vi "Test_Install_IPK.vi"(4 "error in":errorcluster, 7 "Parameter Array in":string[](array[string])) -> (0 "error out":errorcluster, 1 "Result Paragraphs":string[](array[string]), 2 "Pass":bool, 3 "Parameter Array Out":string[](array[string]))   [LabVIEW 2020]
uses:
  <vilib>/nisyscfg/Software 1.2.ctl
  <vilib>/nisyscfg/Component Type.ctl
  CommonSubVIs/Framework/Flattened_Array/Test Parameter Enum.ctl
  CommonSubVIs/Framework/Flattened_Array/Get Parameter Value by Name (String).vi
  <vilib>/nisyscfg/Get Installed Components.vi
  <vilib>/nisyscfg/Close (System).vi
  <resource>/objmgr/nisysapi.rc
  <vilib>/nisyscfg/nisyscfg.lvlib
panel:
  out "Greenways\nBoolean":bool
  in  "Tab Control":T1(tab)
  in  "Network Address":string="10.0.62.162"
  out "Format Python result":string
  out "Format Return Code":i32
  out "Format\nBoolean":bool
  out "Setup Python result":string
  out "Setup Return Code":i32
  out "Setup\nBoolean":bool
  out "GreenWays Python result":string
  out "Greenways Return Code":i32
  out "Installed Software 1":T2[](array[typedef]) caption="Installed Software" {"component type" items=["standard", "hidden", "system", "unknown", "startup", "image", "essential"]}
  # "This VI is used to Format For IPK installation Using python script."
  # "This VI is used to install SetupLinux for RT IPK  Using python script."
  # "This VI is used to install Greenway and FTP software to the (IPK) Linux target Using python script."
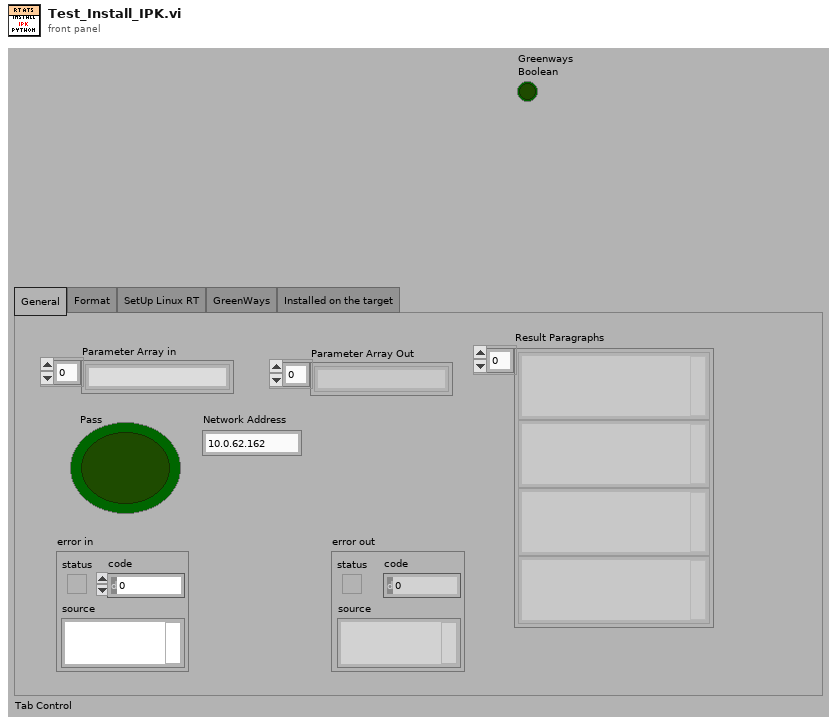
[diagram p1: front panel]
types:
  T1 = enum32{"General", "Format", "SetUp Linux RT", "GreenWays", "Installed on the target"}
  T2 = typedef "nisyscfg.lvlib/Software 1.2.ctl" = cluster{"title":string, "description":string, "ID":string, "version":string, "component type":T3}
  T3 = typedef "nisyscfg.lvlib/Component Type.ctl" = u32
  T4 = typedef "Test Parameter Enum.ctl" = enum16{"Main Test Target IP", "Main Test Target Name", "Main Test Target Alias", "Main Host IP", "Default Target Alias", "Default Target Host Name", "Dafault Target IP Address", "Dafault Target LV Date", "Available Targets", "Target Alias by Index", "Target IP by Alias", "Target IP by  Index", "Current Iteration", "Total Iterations", "Test Project Name", "Current Test Result", "Current Test Name", "Current Test Logical Path", "Test Folder", "Configuration Name", "Configuration Index", "Total Configurations", "Performance Values", "Result Paragraphs", "Connector Pane", "Avoid?", "Avoid Reason", "Case Name", "Case #", "Total Cases", "Case Data", "Disable reason"}
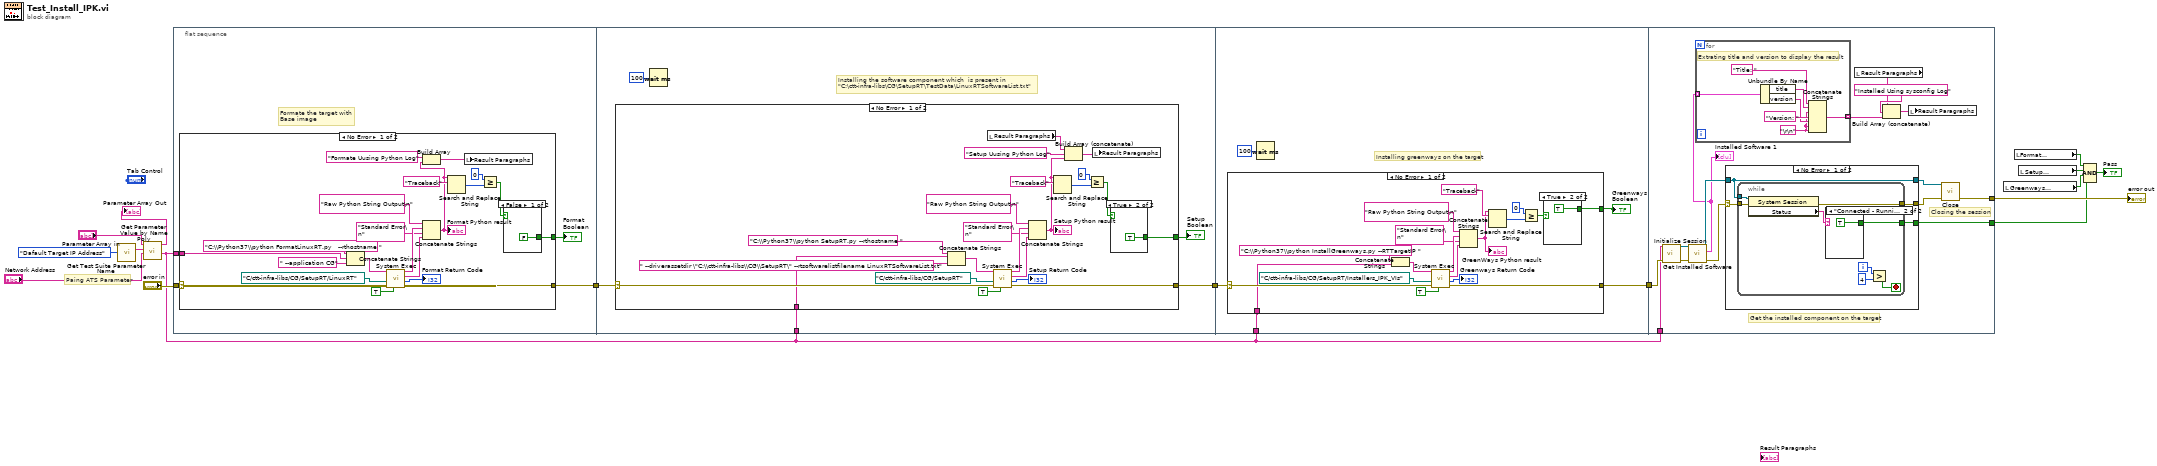
[diagram p0: block diagram]
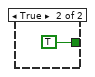
[diagram p2: hidden frame]
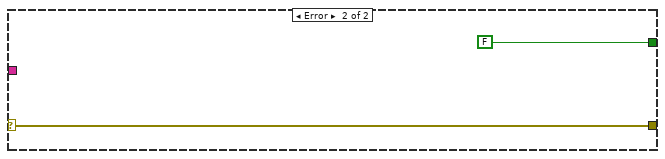
[diagram p3: hidden frame]
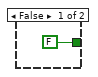
[diagram p4: hidden frame]
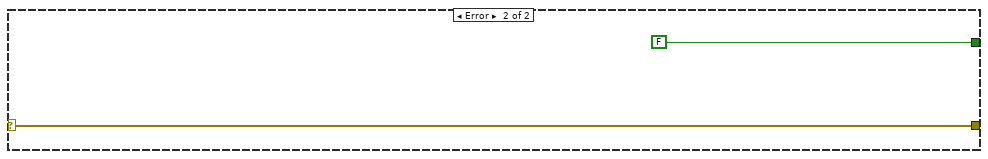
[diagram p5: hidden frame]
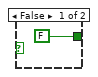
[diagram p6: hidden frame]
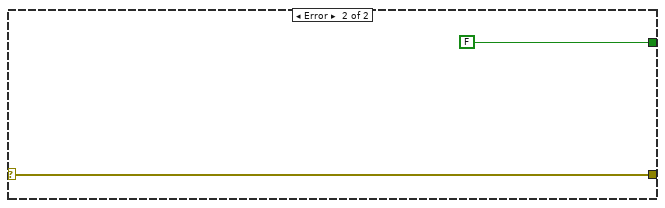
[diagram p7: hidden frame]
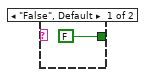
[diagram p8: hidden frame]
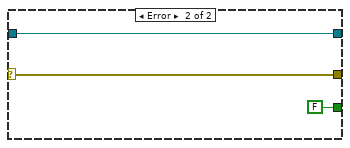
[diagram p9: hidden frame]
diagram:
  # "Paing ATS Parameter"
  n1 = call "Get Test Suite Parameter Name.vi"("Test Suite Parameter"=Test_Parameter_Enum."Dafault Target IP Address") -> ("Parameter Name"=w14:string)  [unwired: 13 in, 1 out]
  n2 = call-poly "Get Parameter Value by Name Poly.vi"("Default Value"="Network Address", "Parameter"=w14, "Parameter Array in"="Parameter Array in") -> ("Value"=w1:string, "Parameter Array Out"=→"Parameter Array Out":string[])  [unwired: 5 in, 1 out]
  n3 = flat-sequence {
    tunnel: "error in" -> [w19]
    tunnel: w1 -> [w18]
    tunnel: [w17] -> w10
    tunnel: w10 -> [w50]
    tunnel: [w49] -> w9
    tunnel: w1 -> [w48]
    tunnel: w9 -> [w81]
    tunnel: w1 -> [w80]
    tunnel: [w79] -> w8
    tunnel: w8 -> [w115]
    tunnel: [w116] -> w7
    tunnel: [w114] -> w6
    tunnel: w1 -> [w109]
    frame #0 {
      # "Formate the target with \nBase image"
      n4 = case shown="No Error" w19 {
        selector: w19 -> [w35 w44]
        tunnel: [w26 FALSE] -> w20
        tunnel: [w34 w44] -> w17
        tunnel: w18 -> [w36 _]
        frame No Error {
          n5 = Concatenate Strings("C:\\Python37\\python FormatLinuxRT.py   --rthostname ", w36, " --application CG" ("string")) -> (w41:string)
          n6 = call <vilib>:"System Exec.vi"("run minimized? (F)"=TRUE, "error in (no error)"=w35, "working directory"=path "C:/ctt-infra-libs/CG/SetupRT/LinuxRT", "command line"=w41) -> ("error out"=w34:errorcluster, "return code"=→"Format Return Code":i32, "standard error"=w29:string, "standard output"=w31:string)  [unwired: 4 in]
          n7 = Concatenate Strings("Raw Python String Output\n" ("string"), w31, "Standard Error\n" ("string 2"), w29) -> (w22:string)
          "Format Python result" <- w22
          n8 = Build Array("Formate Uusing Python Log" ("element"), w22) -> (w23:string[])
          n9 = Search and Replace String(input string=w22, search string="Traceback") -> (number of replacements=w24:i32)  [unwired: 6 in, 3 out]
          n10 = local write "Result Paragraphs"(w23) -> ()
          n11 = Greater Or Equal?(x=0 ("y"), y=w24) -> (x >= y?=w27:bool)
          n12 = case shown="False" w27 {
            tunnel: [FALSE TRUE] -> w26
            frame False {
            }
            frame True {
            }
          }
        }
        frame Error {
        }
      }
      "Format\nBoolean" <- w20
    }
    frame #1 {
      # "Installing the software component which  is present in\n\"C:\\ctt-infra-libs\\CG\\SetupRT\\TestData\\LinuxRTSoftwareList.txt\""
      n13 = case shown="No Error" w50 {
        selector: w50 -> [w67 w75]
        tunnel: [w65 FALSE] -> w47
        tunnel: [w66 w75] -> w49
        tunnel: w48 -> [w55 _]
        frame No Error {
          n14 = Concatenate Strings("C:\\Python37\\python SetupRT.py --rthostname ", w55, " --driverassetdir \"C:\\ctt-infra-libs\\CG\\SetupRT\" --rtsoftwarelistfilename LinuxRTSoftwareList.txt" ("string")) -> (w72:string)
          n15 = local read "Result Paragraphs"() -> (w54:string[])
          n16 = call <vilib>:"System Exec.vi"("run minimized? (F)"=TRUE, "error in (no error)"=w67, "working directory"=path "C:/ctt-infra-libs/CG/SetupRT", "command line"=w72) -> ("error out"=w66:errorcluster, "return code"=→"Setup Return Code":i32, "standard error"=w60:string, "standard output"=w62:string)  [unwired: 4 in]
          n17 = Concatenate Strings("Raw Python String Output\n" ("string"), w62, "Standard Error\n" ("string 2"), w60) -> (w51:string)
          "Setup Python result" <- w51
          n18 = Search and Replace String(input string=w51, search string="Traceback") -> (number of replacements=w57:i32)  [unwired: 6 in, 3 out]
          n19 = Build Array (concatenate)(w54, "Setup Uusing Python Log" ("string"), w51) -> (w52:string[])
          n20 = Greater Or Equal?(x=0 ("y"), y=w57) -> (x >= y?=w56:bool)
          n21 = local write "Result Paragraphs"(w52) -> ()
          n22 = case shown="True" w56 {
            tunnel: [FALSE TRUE] -> w65
            frame False {
            }
            frame True {
            }
          }
        }
        frame Error {
        }
      }
      "Setup\nBoolean" <- w47
      n23 = Wait (ms)(milliseconds to wait=u32 100) -> ()  [unwired: 1 out]
    }
    frame #2 {
      # "Installing greenways on the target"
      n24 = case shown="No Error" w81 {
        selector: w81 -> [w94 w103]
        tunnel: [w93 w103] -> w79
        tunnel: [w83 FALSE] -> w78
        tunnel: w80 -> [w82 _]
        frame No Error {
          n25 = Concatenate Strings("C:\\Python37\\python InstallGreenways.py --RTTargetIP ", w82) -> (w99:string)
          n26 = call <vilib>:"System Exec.vi"("run minimized? (F)"=TRUE, "error in (no error)"=w94, "working directory"=path "C:/ctt-infra-libs/CG/SetupRT/Installers_IPK_VIs", "command line"=w99) -> ("error out"=w93:errorcluster, "return code"=→"Greenways Return Code":i32, "standard error"=w92:string, "standard output"=w91:string)  [unwired: 4 in]
          n27 = Concatenate Strings("Raw Python String Output\n" ("string"), w91, "Standard Error\n" ("string 2"), w92) -> (w84:string)
          "GreenWays Python result" <- w84
          n28 = Search and Replace String(input string=w84, search string="Traceback") -> (number of replacements=w88:i32)  [unwired: 6 in, 3 out]
          n29 = Greater Or Equal?(x=0 ("y"), y=w88) -> (x >= y?=w87:bool)
          n30 = case shown="True" w87 {
            tunnel: [FALSE TRUE] -> w83
            frame False {
            }
            frame True {
            }
          }
        }
        frame Error {
        }
      }
      "Greenways\nBoolean" <- w78
      n31 = Wait (ms)(milliseconds to wait=u32 100) -> ()  [unwired: 1 out]
    }
    frame #3 {
      # "Get the installed component on the target"
      # "Closing the session"
      n32 = call <vilib>:"Initialize Session.vi"("error in (no error)"=w115, "Target (localhost)"=w109) -> ("error out"=w104:errorcluster, "Session out"=w108:refnum<k21>)  [unwired: 8 in]
      n33 = call-poly <vilib>:"Get Installed Software.vi"("error in (no error)"=w104, "Session in"=w108) -> ("error out"=w105:errorcluster, "Software Components"=w106:T2[], "Session out"=w107:refnum<k21>)  [unwired: 7 in]
      "Installed Software 1" <- w106
      n34 = for {
        tunnel: w106 -> [w125] mode=indexing
        tunnel: [w120] -> w112 mode=indexing
        w119 = "\r\n"
        # "Extrating title and version to display the result"
        n35 = Unbundle By Name(w125) -> ("title"=w123:string, "version"=w121:string)
        n36 = Concatenate Strings("Title: " ("string"), w123, w119, "Version: " ("string"), w121, w119, w119) -> (w120:string)
      }
      n37 = case shown="No Error" w105 {
        selector: w105 -> [w128 w140]
        tunnel: w107 -> [w126 w142]
        tunnel: [w129 FALSE] -> w114
        tunnel: [w126 w142] -> w117
        tunnel: [w127 w140] -> w118
        frame No Error {
          n38 = while {
            tunnel: w128 -> [w133]
            tunnel: [w130] -> w127
            tunnel: [w137] -> w129
            tunnel: w126 -> [w132]
            i -> [w136]
            stop <- w134 stop-if-true
            n39 = property class="System Session"(reference=w132, error in=w133) -> (error out=w130:errorcluster, "Status"=w131:string)  [unwired: 1 out]
            n40 = case shown="\"Connected - Running\"" w131 {
              tunnel: [FALSE TRUE] -> w137
              frame "False", Default {
              }
              frame "Connected - Running" {
              }
            }
            n41 = Greater?(x=w136, y=4) -> (0:w134:bool)
          }
        }
        frame Error {
        }
      }
      n42 = local read "Result Paragraphs"() -> (w110:string[])
      n43 = Build Array (concatenate)(w110, "Installed Using sysconfig Log" ("string"), w112) -> (w111:string[])
      n44 = local write "Result Paragraphs"(w111) -> ()
      n45 = call-poly <vilib>:"Close.vi"("error in (no error)"=w118, "Session in"=w117) -> ("error out"=w116:errorcluster)  [unwired: 9 in]
    }
  }
  n46 = local read "Greenways\nBoolean"() -> (w4:bool)
  n47 = local read "Format\nBoolean"() -> (w2:bool)
  n48 = local read "Setup\nBoolean"() -> (w3:bool)
  n49 = Compound Arithmetic op=AND(w2, w3, w4, w6) -> (→"Pass":bool)
  "error out" <- w7
